vi "MH_DllPath_global.vi"() -> ()   [LabVIEW 2019]
panel:
  in  "DllPath":path=path "C:/Windows/System32/mhlib64.dll"
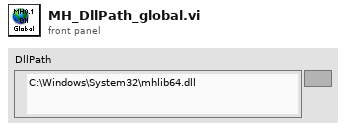
[diagram p1: front panel]
diagram:
